vi "3D-AnalystROIArray.vi"(0 "Pic Param  Data Collect":string[][](table)=[["", "", ""], ["", "", ""]]) -> (14 "ALabelArray":string[](array[string]), 15 "BLabelArray":string[](array[string]), 16 "StepNameA":string[](array[string]), 17 "StepNameB":string[](array[string]), 18 "TeatNameA":string[](array[string]), 19 "TestNameB":string[](array[string]), 20 "A ROI Array":dbl[][](array[numeric]), 21 "A USL":cluster{"USL":dbl, "LSL":dbl}[](array[cluster]), 23 "A ROI Array":T1[](array[typedef]) {"Rotation" format="%.2f"; "Left" scale=0.0..1024.0; "Right" scale=0.0..1024.0}, 24 "B ROI Array":T1[](array[typedef]) {"Rotation" format="%.2f"; "Left" scale=0.0..1024.0; "Right" scale=0.0..1024.0}, 25 "B USL":cluster{"USL":dbl, "LSL":dbl}[](array[cluster]), 27 "B ROI Array":dbl[][](array[numeric]))   [LabVIEW 2015]
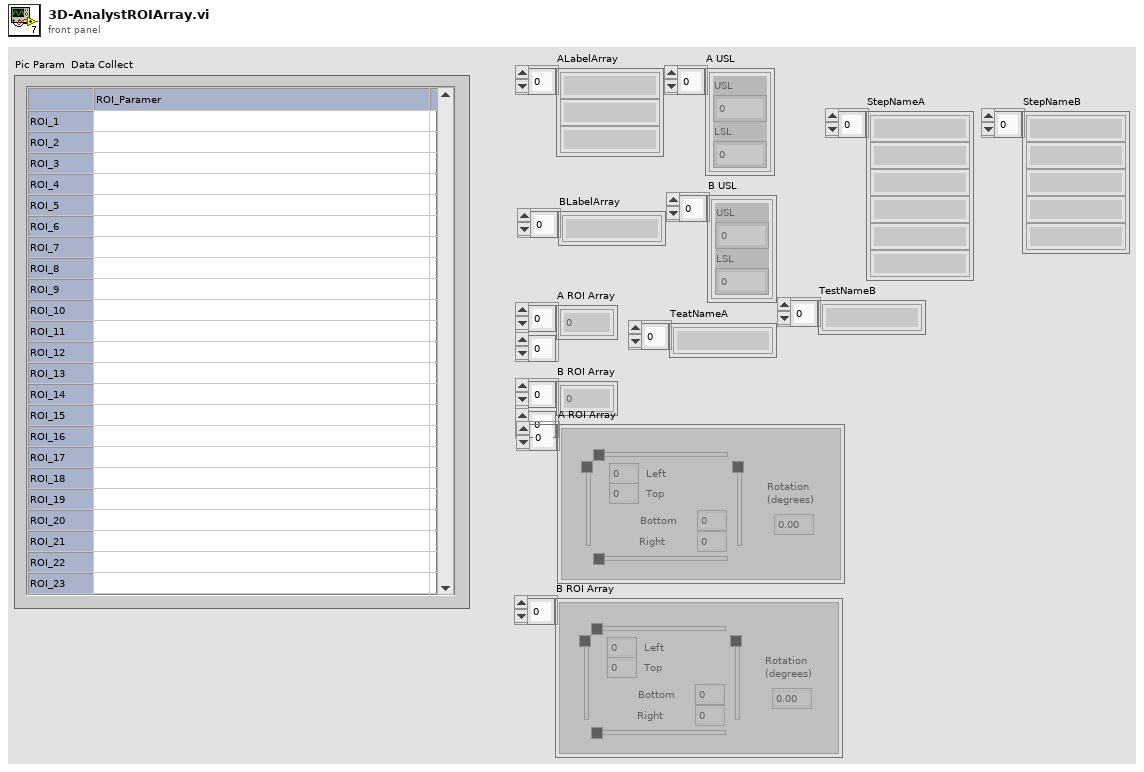
[diagram p1: front panel]
types:
  T1 = typedef "IMAQ Rectangle" = cluster{"Left":i32, "Top":i32, "Right":i32, "Bottom":i32, "Rotation":dbl}
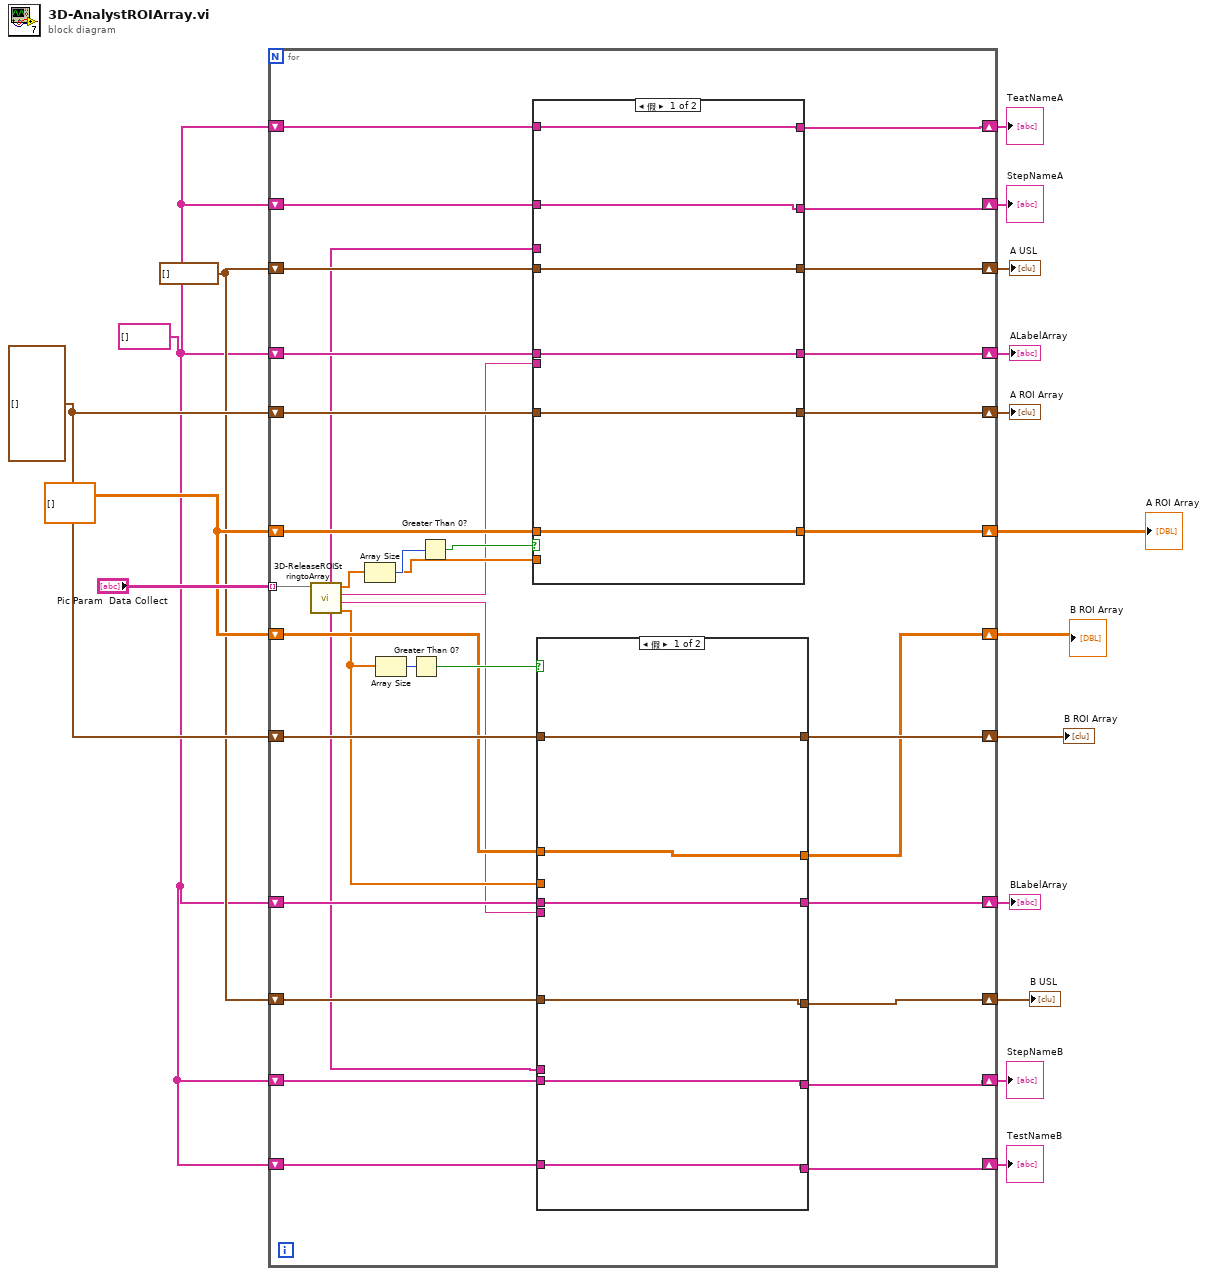
[diagram p0: block diagram]
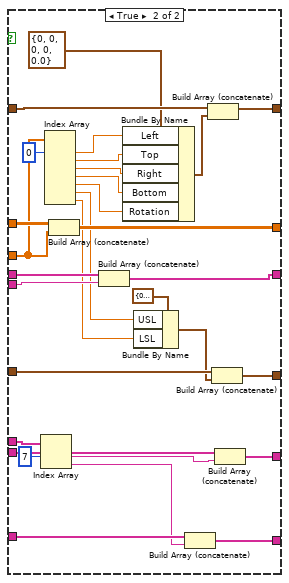
[diagram p2: hidden frame]
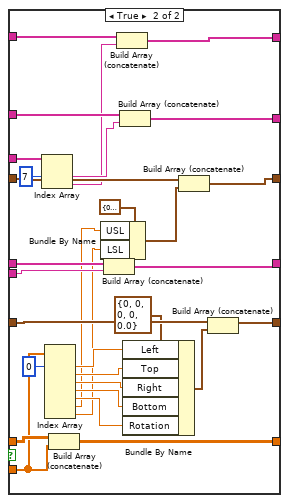
[diagram p3: hidden frame]
diagram:
  w8 = cluster{"USL":dbl, "LSL":dbl}[] []
  w2 = string[] []
  w13 = T1[] []
  w16 = dbl[][] []
  n1 = for {
    tunnel: "Pic Param  Data Collect" -> [w52] mode=indexing
    shift-right: [w47] -> w15
    shift-left: w16 -> [w49]
    shift-right: [w39] -> w14
    shift-left: w16 -> [w40]
    shift-right: [w44] -> w12
    shift-left: w13 -> [w45]
    shift-right: [w42] -> w11
    shift-left: w13 -> [w43]
    shift-right: [w36] -> w10
    shift-left: w2 -> [w37]
    shift-right: [w34] -> w9
    shift-left: w2 -> [w35]
    shift-right: [w30] -> w7
    shift-left: w8 -> [w31]
    shift-right: [w28] -> w6
    shift-left: w8 -> [w29]
    shift-right: [w25] -> w5
    shift-left: w2 -> [w26]
    shift-right: [w23] -> w4
    shift-left: w2 -> [w24]
    shift-right: [w20] -> w3
    shift-left: w2 -> [w21]
    shift-right: [w18] -> w1
    shift-left: w2 -> [w19]
    n2 = call "3D-ReleaseROIStringtoArray.vi"("ROI Information"=w52) -> (0:"B ROI Param"=w38:dbl[], "B_label"=w32:string, "A_label"=w33:string, 3:"A ROI Param"=w48:dbl[], 4:"B ROI Param"=w22:string[], 5:"A ROI Param"=w27:string[])  [unwired: 5 in]
    n3 = Array Size(array=w48) -> (size(s)=w51:i32)
    n4 = Array Size(array=w38) -> (size(s)=w46:i32)
    n5 = Greater Than 0?(x=w46) -> (x > 0?=w41:bool)
    n6 = Greater Than 0?(x=w51) -> (x > 0?=w50:bool)
    n7 = case shown="假" w50 {
      tunnel: w49 -> [w94 w124]
      tunnel: w48 -> [_ w118]
      tunnel: [w94 w123] -> w47
      tunnel: w45 -> [w93 w122]
      tunnel: [w93 w121] -> w44
      tunnel: w37 -> [w92 w111]
      tunnel: [w92 w110] -> w36
      tunnel: w33 -> [_ w109]
      tunnel: w31 -> [w91 w105]
      tunnel: [w91 w104] -> w30
      tunnel: w27 -> [_ w100]
      tunnel: w26 -> [w90 w102]
      tunnel: [w90 w101] -> w25
      tunnel: w21 -> [w89 w97]
      tunnel: [w89 w95] -> w20
      frame False {
      }
      frame True {
        n8 = Index Array(array=w100, index #1=7 ("索引")) -> (element #1=w98:string, element #2=w96:string)  [unwired: 1 in]
        n9 = Index Array(array=w118, index #1=0 ("索引")) -> (element #1=w116:dbl, element #2=w115:dbl, element #3=w114:dbl, element #4=w113:dbl, element #5=w112:dbl, element #6=w107:dbl, element #7=w106:dbl)  [unwired: 6 in]
        n10 = Build Array (concatenate)(w124, w118) -> (w123:dbl[][])
        n11 = Bundle By Name(cluster=cluster{"USL":dbl, "LSL":dbl} {"USL"=0.0, "LSL"=0.0}, "USL"=w107, "LSL"=w106) -> (w103:cluster{"USL":dbl, "LSL":dbl})
        n12 = Build Array (concatenate)(w111, w109) -> (w110:string[])
        n13 = Build Array (concatenate)(w97, w96) -> (w95:string[])
        n14 = Build Array (concatenate)(w102, w98) -> (w101:string[])
        n15 = Bundle By Name(cluster=T1 {"Left"=0, "Top"=0, "Right"=0, "Bottom"=0, "Rotation"=0.0} ("Rectangle"), "Left"=w116, "Top"=w115, "Right"=w114, "Bottom"=w113, "Rotation"=w112) -> (w119:T1)
        n16 = Build Array (concatenate)(w105, w103) -> (w104:cluster{"USL":dbl, "LSL":dbl}[])
        n17 = Build Array (concatenate)(w122, w119) -> (w121:T1[])
      }
    }
    n18 = case shown="假" w41 {
      tunnel: w40 -> [w58 w88]
      tunnel: [w58 w87] -> w39
      tunnel: w43 -> [w57 w86]
      tunnel: [w57 w85] -> w42
      tunnel: w38 -> [_ w76]
      tunnel: w35 -> [w56 w75]
      tunnel: [w56 w73] -> w34
      tunnel: w32 -> [_ w74]
      tunnel: w29 -> [w55 w71]
      tunnel: [w55 w70] -> w28
      tunnel: w24 -> [w54 w66]
      tunnel: [w54 w65] -> w23
      tunnel: w22 -> [_ w64]
      tunnel: w19 -> [w53 w61]
      tunnel: [w53 w60] -> w18
      frame False {
      }
      frame True {
        n19 = Index Array(array=w64, index #1=7 ("索引")) -> (element #1=w62:string, element #2=w59:string)  [unwired: 1 in]
        n20 = Index Array(array=w76, index #1=0 ("索引")) -> (element #1=w81:dbl, element #2=w80:dbl, element #3=w79:dbl, element #4=w78:dbl, element #5=w77:dbl, element #6=w68:dbl, element #7=w67:dbl)  [unwired: 6 in]
        n21 = Build Array (concatenate)(w88, w76) -> (w87:dbl[][])
        n22 = Build Array (concatenate)(w75, w74) -> (w73:string[])
        n23 = Bundle By Name(cluster=T1 {"Left"=0, "Top"=0, "Right"=0, "Bottom"=0, "Rotation"=0.0} ("Rectangle"), "Left"=w81, "Top"=w80, "Right"=w79, "Bottom"=w78, "Rotation"=w77) -> (w83:T1)
        n24 = Bundle By Name(cluster=cluster{"USL":dbl, "LSL":dbl} {"USL"=0.0, "LSL"=0.0}, "USL"=w68, "LSL"=w67) -> (w69:cluster{"USL":dbl, "LSL":dbl})
        n25 = Build Array (concatenate)(w61, w59) -> (w60:string[])
        n26 = Build Array (concatenate)(w86, w83) -> (w85:T1[])
        n27 = Build Array (concatenate)(w71, w69) -> (w70:cluster{"USL":dbl, "LSL":dbl}[])
        n28 = Build Array (concatenate)(w66, w62) -> (w65:string[])
      }
    }
  }
  "A ROI Array" <- w15
  "B ROI Array" <- w14
  "A ROI Array" <- w12
  "B ROI Array" <- w11
  "ALabelArray" <- w10
  "BLabelArray" <- w9
  "A USL" <- w7
  "B USL" <- w6
  "StepNameA" <- w5
  "StepNameB" <- w4
  "TeatNameA" <- w3
  "TestNameB" <- w1
